vi "niTuner Set Freq(f).vi"(8 "error in":errorcluster, 9 "span":dbl=20000000.0 format="%.2p", 10 "desired RF frequency":dbl format="%.2f", 11 "taskID in":i32 format="%.0x") -> (0 "error out":errorcluster, 1 "actual RF tuned frequency":dbl format="%.2f", 2 "actual IF frequency":dbl format="%.2f", 3 "taskID out":i32 format="%.0x", 4 "frequency shift":dbl format="%.2f")   [LabVIEW 2011]
doc: "This instance of the polymorphic VI sets a single center frequency in the scan list and immediately begins to settle on that frequency.\n\nNOTE: If new center frequencies of less than 15 MHz are specified by a call to this VI, attenuation may be automatically adjusted. This may add up to an additional 20 dB attenuation."
uses:
  nipxi5600u.dll
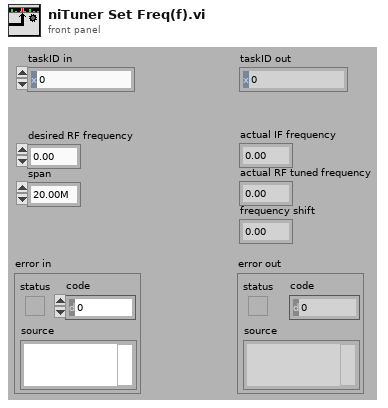
[diagram p1: front panel]
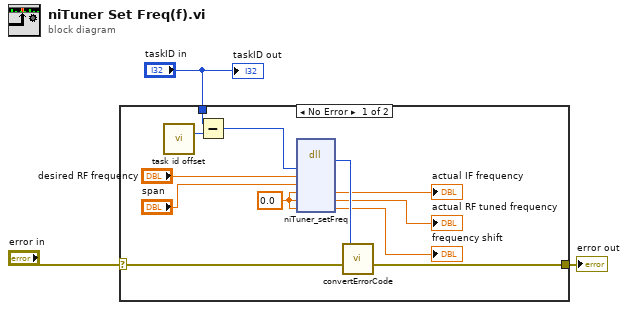
[diagram p0: block diagram]
diagram:
  n1 = case shown="No Error" "error in" {
    selector: "error in" -> [w14 w16]
    tunnel: [w13 w16] -> w2
    tunnel: "taskID in" -> [w6 _]
    frame No Error {
      w7 = 0.0 ("actualIFCenterFrequency")
      n2 = call <instrlib>:"task id offset.vi"() -> ("taskID offset"=w5:i32)
      n3 = Subtract(x=w6, y=w5) -> (x-y=w4:i32)
      n4 = dll-call lib="nipxi5600u.dll" fn="niTuner_setFreq"("taskID"=w4, "desiredRFCenterFrequency"="desired RF frequency", "span"="span", "actualIFCenterFrequency"=w7, "actualRFCenterFrequency"=w7, "freqShift"=w7) -> (w15:i32, "actualIFCenterFrequency"=→"actual IF frequency":dbl, "actualRFCenterFrequency"=→"actual RF tuned frequency":dbl, "freqShift"=→"frequency shift":dbl)  [unwired: 6 in, 2 out]
      n5 = call <instrlib>:"convertErrorCode.vi"("error in"=w14, "error code"=w15) -> ("error out"=w13:errorcluster)
    }
    frame Error {
    }
  }
  "error out" <- w2
  "taskID out" <- "taskID in"
